vi "populateEventHardpointActuatorInfo.vi"(8 "error in (no error)":errorcluster, 11 "Model in":refnum<class "Model.lvclass">) -> (0 "error out":errorcluster, 3 "Model out":refnum<class "Model.lvclass">)   [LabVIEW 2016, in "Model.lvclass"]
uses:
  Model.lvclass
  Model.lvclass/Model.ctl
  ILCCommunications/ILCCommunications.lvclass/ILCCommunications.ctl
  Publisher/Publisher.lvclass/Publisher.ctl
  Common_RT_HPILC/HPILC/HPILC.lvclass/HPILC.ctl
  Common_RT_ILC/ILC/ILC.lvclass/ILC.ctl
  Common_RT_HPILC/HPILC/HPILC.lvclass
  D:/Code/ts_M1M3Support/Common_RT_ILC/ILC/ILC.lvclass
  ILCCommunications/ILCCommunications.lvclass
  Publisher/Publisher.lvclass
  Common_RT_ILC/ILC/ILC.lvclass
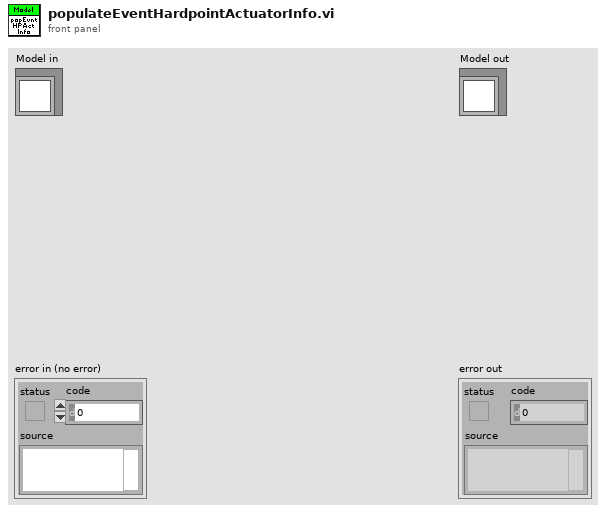
[diagram p1: front panel]
types:
  T1 = typedef "RTILC.lvlib/ILCData.ctl" = cluster{"Constants":T2, "Command":T3, "Telemetry":T5, "Responses":T6, "Timings":T8}
  T2 = typedef "RTILC.lvlib/ILCConstants.ctl" = cluster{"Subnet":u8, "Address":u8}
  T3 = typedef "RTILC.lvlib/ILCCommand.ctl" = cluster{"ILCMode":u16, "TemporaryAddress":u8, "ADCScanRate":T4, "ADCChannel":u8, "ADCOffset":sgl, "ADCSensitivity":sgl}
  T4 = typedef "RTILC.lvlib/ILCScanRates.ctl" = u8
  T5 = typedef "RTILC.lvlib/ILCTelemetry.ctl" = cluster{"UniqueID":u64, "FirmwareType":u8, "NetworkNodeType":u8, "ILCOption":u8, "NetworkNodeOption":u8, "MajorRevision":u8, "MinorRevision":u8, "FirmwareName":string, "ILCMode":u16, "MajorFault":bool, "MinorFault":bool, "FaultOverride":bool, "MainCalibrationError":bool, "BackupCalibrationError":bool, "UniqueIDCRCMismatch":bool, "AppTypeNodeTypeMismatch":bool, "AppMissing":bool, "AppCRCMismatch":bool, "TEDSNotFound":bool, "TEDS1Mismatch":bool, "TEDS2Mismatch":bool, "WatchdogResetDetected":bool, "BrownoutDetected":bool, "EventTrapResetDetected":bool, "MotorPowerFault":bool, "SSRPowerFault":bool, "AuxPowerFault":bool, "SMCPowerFault":bool, "TemporaryAddress":u8, "ADCScanRate":T4, "DAC1":u16, "DAC2":u16, "DAC3":u16, "DAC4":u16, "MainADCCalibrationK":sgl[], "MainSensorOffset":sgl[], "MainSensorSensitivity":sgl[], "BackupADCCalibrationK":sgl[], "BackupSensorOffset":sgl[], "BackupSensorSensitivity":sgl[]}
  T6 = typedef "RTILC.lvlib/ILCResponses.ctl" = cluster{"ReportServerID":T7, "ReportServerStatus":T7, "ILCMode":T7, "SetTemporaryAddress":T7, "Reset":T7, "ADCScanRate":T7, "ADCOffsetSensitivity":T7, "ReadDAC":T7, "ReadCalibration":T7}
  T7 = typedef "RTModbus.lvlib/ExceptionCodes.ctl" = u16
  T8 = typedef "RTILC.lvlib/ILCTimings.ctl" = cluster{"ADCOffsetSensitivity":u32, "ADCScanRate":u32, "ILCMode":u32, "ReadCalibration":u32, "ReportServerID":u32, "ReportServerStatus":u32, "Reset":u32, "SetTemporaryAddress":u32}
  T9 = typedef "RTHPILC.lvlib/HPData.ctl" = cluster{"Constants":T10, "Command":T11, "Telemetry":T12, "Responses":T13, "Timings":T14}
  T10 = typedef "RTHPILC.lvlib/HPConstants.ctl" = cluster{"ID":i16, "ReferencePosition":i32, "XPosition":sgl, "YPosition":sgl, "ZPosition":sgl}
  T11 = typedef "RTHPILC.lvlib/HPCommand.ctl" = cluster{"Steps":i8}
  T12 = typedef "RTHPILC.lvlib/HPTelemetry.ctl" = cluster{"ILCFault":bool, "LimitSwitchCWOperated":bool, "LimitSwitchCCWOperated":bool, "BroadcastCounter":u8, "SSIEncoderValue":i32, "LoadCellForce":sgl}
  T13 = typedef "RTHPILC.lvlib/HPResponses.ctl" = cluster{"StepMotor":T7, "ForceAndStatus":T7}
  T14 = typedef "RTHPILC.lvlib/HPTimings.ctl" = cluster{"BroadcastStepMotor":u32, "ForceAndStatus":u32, "FreezeSensorValues":u32, "StepMotor":u32}
  T15 = typedef "M1M3SupportTopics.lvlib/Timestamp.ctl" = dbl
  T16 = typedef "M1M3SupportTopics.lvlib/EventHardpointActuatorInfo.ctl" = cluster{"Timestamp":T15, "ReferenceId":i32[], "ReferencePosition":i32[], "XPosition":sgl[], "YPosition":sgl[], "ZPosition":sgl[], "ILCUniqueId":i64[], "ILCApplicationType":u8[], "NetworkNodeType":u8[], "ILCSelectedOptions":u8[], "NetworkNodeOptions":u8[], "MajorRevision":u8[], "MinorRevision":u8[], "ADCScanRate":u8[], "MainADCCalibrationK1":sgl[], "MainADCCalibrationK2":sgl[], "MainADCCalibrationK3":sgl[], "MainADCCalibrationK4":sgl[], "MainLoadCellOffset":sgl[], "MainLoadCellSensitivity":sgl[], "BackupADCCalibrationK1":sgl[], "BackupADCCalibrationK2":sgl[], "BackupADCCalibrationK3":sgl[], "BackupADCCalibrationK4":sgl[], "BackupLoadCellOffset":sgl[], "BackupLoadCellSensitivity":sgl[], "MainCalibrationError":bool[], "BackupCalibrationError":bool[], "UniqueIdCRCError":bool[], "ApplicationTypeMismatch":bool[], "ApplicationMissing":bool[], "ApplicationCRCMismatch":bool[], "OneWireMissing":bool[], "OneWire1Mismatch":bool[], "OneWire2Mismatch":bool[]}
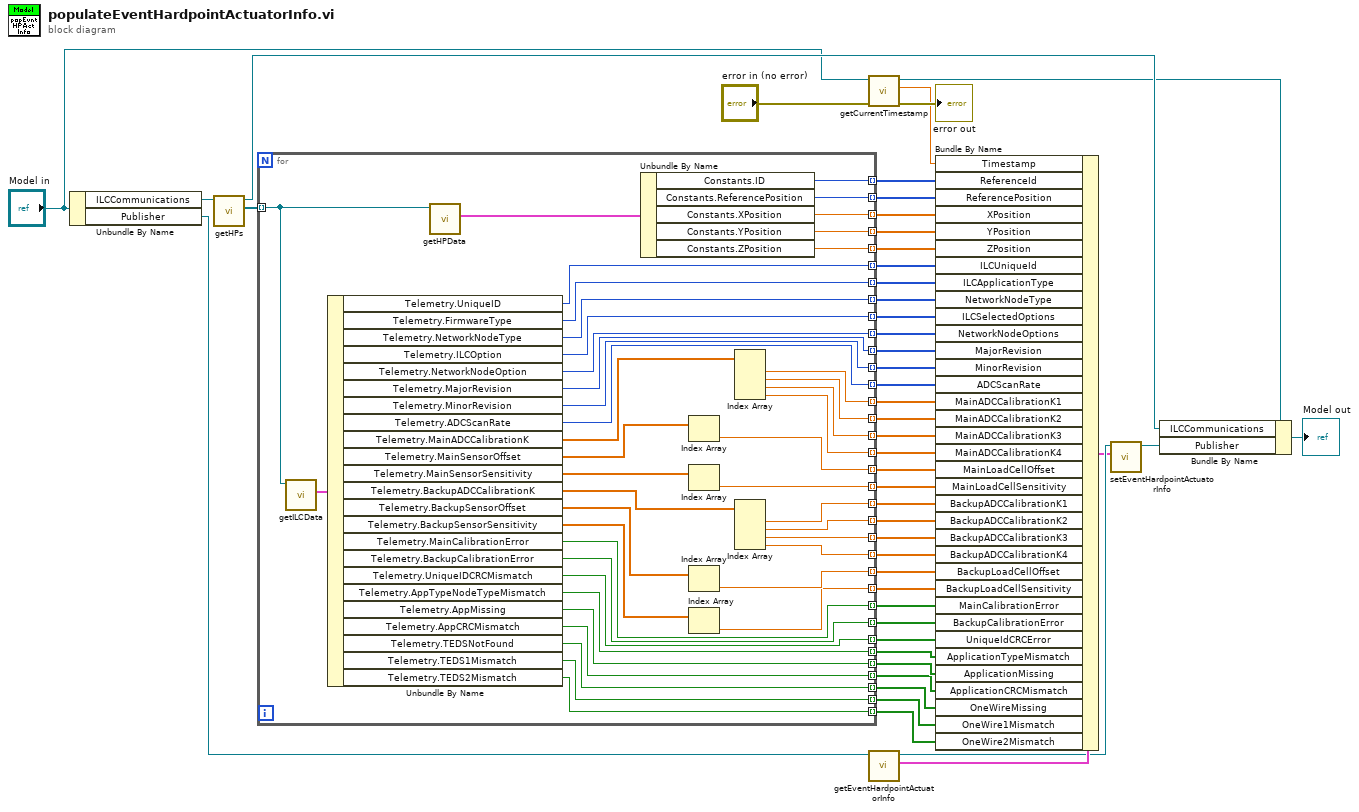
[diagram p0: block diagram]
diagram:
  n1 = Unbundle By Name("Model in") -> ("ILCCommunications"=w47:refnum<class "ILCCommunications.lvclass">, "Publisher"=w46:refnum<class "Publisher.lvclass">)
  n2 = call "getHPs.vi"("ILCCommunications in"=w47) -> ("HPs"=w42:refnum<class "HPILC.lvclass">[], "ILCCommunications out"=w10:refnum<class "ILCCommunications.lvclass">)  [unwired: 9 in]
  n3 = for {
    tunnel: w42 -> [w55] mode=indexing
    tunnel: [w89] -> w41 mode=indexing
    tunnel: [w88] -> w40 mode=indexing
    tunnel: [w87] -> w39 mode=indexing
    tunnel: [w86] -> w38 mode=indexing
    tunnel: [w85] -> w37 mode=indexing
    tunnel: [w84] -> w36 mode=indexing
    tunnel: [w83] -> w35 mode=indexing
    tunnel: [w82] -> w34 mode=indexing
    tunnel: [w81] -> w33 mode=indexing
    tunnel: [w80] -> w32 mode=indexing
    tunnel: [w79] -> w31 mode=indexing
    tunnel: [w78] -> w30 mode=indexing
    tunnel: [w76] -> w29 mode=indexing
    tunnel: [w74] -> w28 mode=indexing
    tunnel: [w72] -> w27 mode=indexing
    tunnel: [w71] -> w26 mode=indexing
    tunnel: [w70] -> w25 mode=indexing
    tunnel: [w69] -> w24 mode=indexing
    tunnel: [w67] -> w23 mode=indexing
    tunnel: [w65] -> w22 mode=indexing
    tunnel: [w64] -> w21 mode=indexing
    tunnel: [w63] -> w20 mode=indexing
    tunnel: [w62] -> w19 mode=indexing
    tunnel: [w61] -> w18 mode=indexing
    tunnel: [w60] -> w17 mode=indexing
    tunnel: [w59] -> w16 mode=indexing
    tunnel: [w58] -> w15 mode=indexing
    tunnel: [w57] -> w14 mode=indexing
    tunnel: [w56] -> w13 mode=indexing
    tunnel: [w53] -> w12 mode=indexing
    tunnel: [w52] -> w4 mode=indexing
    tunnel: [w51] -> w3 mode=indexing
    tunnel: [w50] -> w2 mode=indexing
    tunnel: [w49] -> w1 mode=indexing
    n4 = call "getILCData.vi"("ILC in"=w55) -> ("ILCData"=w91:T1)  [unwired: 9 in, 1 out]
    n5 = Unbundle By Name(w91) -> ("Telemetry.UniqueID"=w89:u64, "Telemetry.FirmwareType"=w88:u8, "Telemetry.NetworkNodeType"=w87:u8, "Telemetry.ILCOption"=w86:u8, "Telemetry.NetworkNodeOption"=w85:u8, "Telemetry.MajorRevision"=w84:u8, "Telemetry.MinorRevision"=w83:u8, "Telemetry.ADCScanRate"=w82:T4, "Telemetry.MainADCCalibrationK"=w90:sgl[], "Telemetry.MainSensorOffset"=w77:sgl[], "Telemetry.MainSensorSensitivity"=w75:sgl[], "Telemetry.BackupADCCalibrationK"=w73:sgl[], "Telemetry.BackupSensorOffset"=w68:sgl[], "Telemetry.BackupSensorSensitivity"=w66:sgl[], "Telemetry.MainCalibrationError"=w64:bool, "Telemetry.BackupCalibrationError"=w63:bool, "Telemetry.UniqueIDCRCMismatch"=w62:bool, "Telemetry.AppTypeNodeTypeMismatch"=w61:bool, "Telemetry.AppMissing"=w60:bool, "Telemetry.AppCRCMismatch"=w59:bool, "Telemetry.TEDSNotFound"=w58:bool, "Telemetry.TEDS1Mismatch"=w57:bool, "Telemetry.TEDS2Mismatch"=w56:bool)
    n6 = call "getHPData.vi"("HPILC in"=w55) -> ("HPData"=w54:T9)  [unwired: 9 in, 1 out]
    n7 = Unbundle By Name(w54) -> ("Constants.ID"=w53:i16, "Constants.ReferencePosition"=w49:i32, "Constants.XPosition"=w52:sgl, "Constants.YPosition"=w51:sgl, "Constants.ZPosition"=w50:sgl)
    n8 = Index Array(array=w77) -> (element=w76:sgl)  [unwired: 1 in]
    n9 = Index Array(array=w75) -> (element=w74:sgl)  [unwired: 1 in]
    n10 = Index Array(array=w68) -> (element=w67:sgl)  [unwired: 1 in]
    n11 = Index Array(array=w66) -> (element=w65:sgl)  [unwired: 1 in]
    n12 = Index Array(array=w90) -> (element #1=w81:sgl, element #2=w80:sgl, element #3=w79:sgl, element #4=w78:sgl)  [unwired: 4 in]
    n13 = Index Array(array=w73) -> (element #1=w72:sgl, element #2=w71:sgl, element #3=w70:sgl, element #4=w69:sgl)  [unwired: 4 in]
  }
  n14 = call "getCurrentTimestamp.vi"("error in (no error)"="error in (no error)", "Model in"="Model in") -> ("error out"=→"error out":errorcluster, "Timestamp"=w5:T15, "Model out"=w8:refnum<class "Model.lvclass">)  [unwired: 7 in]
  n15 = call "getEventHardpointActuatorInfo.vi"("Publisher in"=w46) -> ("EventHardpointActuatorInfo"=w45:T16, "Publisher out"=w44:refnum<class "Publisher.lvclass">)  [unwired: 9 in]
  n16 = Bundle By Name(cluster=w45, "Timestamp"=w5, "ReferenceId"=w12, "ReferencePosition"=w1, "XPosition"=w4, "YPosition"=w3, "ZPosition"=w2, "ILCUniqueId"=w41, "ILCApplicationType"=w40, "NetworkNodeType"=w39, "ILCSelectedOptions"=w38, "NetworkNodeOptions"=w37, "MajorRevision"=w36, "MinorRevision"=w35, "ADCScanRate"=w34, "MainADCCalibrationK1"=w33, "MainADCCalibrationK2"=w32, "MainADCCalibrationK3"=w31, "MainADCCalibrationK4"=w30, "MainLoadCellOffset"=w29, "MainLoadCellSensitivity"=w28, "BackupADCCalibrationK1"=w27, "BackupADCCalibrationK2"=w26, "BackupADCCalibrationK3"=w25, "BackupADCCalibrationK4"=w24, "BackupLoadCellOffset"=w23, "BackupLoadCellSensitivity"=w22, "MainCalibrationError"=w21, "BackupCalibrationError"=w20, "UniqueIdCRCError"=w19, "ApplicationTypeMismatch"=w18, "ApplicationMissing"=w17, "ApplicationCRCMismatch"=w16, "OneWireMissing"=w15, "OneWire1Mismatch"=w14, "OneWire2Mismatch"=w13) -> (w43:T16)
  n17 = call "setEventHardpointActuatorInfo.vi"("EventHardpointActuatorInfo"=w43, "Publisher in"=w44) -> ("Publisher out"=w11:refnum<class "Publisher.lvclass">)  [unwired: 9 in]
  n18 = Bundle By Name(cluster=w8, "ILCCommunications"=w10, "Publisher"=w11) -> (→"Model out":refnum<class "Model.lvclass">)
